vi "emi_Close Loop.vi"   [LabVIEW 2010]
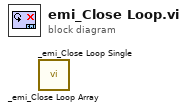
[diagram p0: block diagram]
diagram:
  n1 = call "_emi_Close Loop Array.vi"() -> ()  [unwired: 15 in, 1 out]
  n2 = call "_emi_Close Loop Single.vi"() -> ()  [unwired: 15 in, 1 out]
